vi "Request Joystick State.vi"(8 "error in (no error)":errorcluster, 9 "Caller Enqueuer":refnum<class "Message Enqueuer.lvclass">, 10 "Joystick State Msg":refnum<class "Get Joystick State Msg.lvclass">, 11 "Joystick in":refnum<class "Joystick.lvclass">) -> (0 "error out":errorcluster, 3 "Joystick out":refnum<class "Joystick.lvclass">)   [LabVIEW 2014, in "Joystick.lvlib" / "Joystick.lvclass"]
uses:
  Joystick.lvclass
  Joystick Messages/Get Joystick State Msg/Get Joystick State Msg.lvclass
  <vilib>/ActorFramework/Message Enqueuer/Message Enqueuer.lvclass
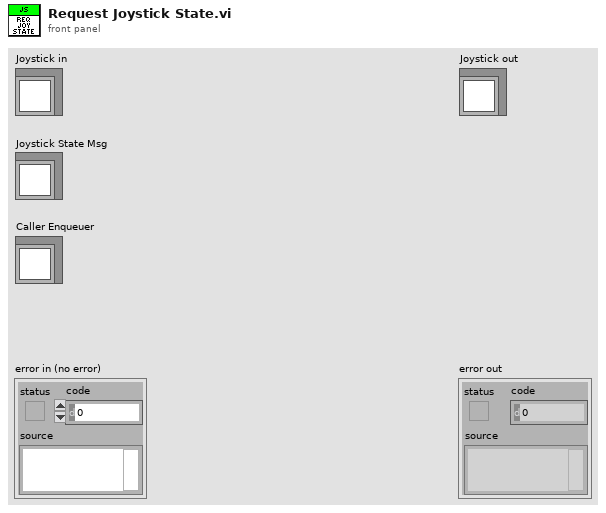
[diagram p1: front panel]
types:
  T1 = typedef "Joystick.lvlib/Joystick.lvclass/Joystick State.ctl" = cluster{"Buttons":T2[], "Axis":T3[]}
  T2 = typedef "Joystick.lvlib/Joystick.lvclass/Button State.ctl" = cluster{"Pressed":bool, "Instance Name":string, "Toggled":bool, "Just Changed":bool}
  T3 = typedef "Joystick.lvlib/Joystick.lvclass/Axis State.ctl" = cluster{"Instance Name":string, "Deadband":dbl, "Value":dbl, "At Home":bool, "Postive Axis Button State":T2, "Negative Axis Button State":T2, "Home Axis Button State":T2}
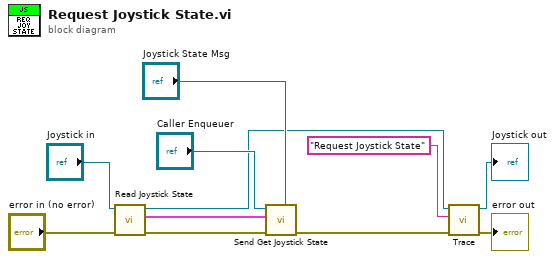
[diagram p0: block diagram]
diagram:
  n1 = call-dynamic "Read Joystick State.vi"("error in (no error)"="error in (no error)", "Joystick in"="Joystick in") -> ("error out"=w8:errorcluster, "Joystick State"=w9:T1, "Joystick out"=w3:refnum<class "Joystick.lvclass">)  [unwired: 7 in]
  n2 = call "Send Get Joystick State.vi"("Joystick.lvlib:Get Joystick State Msg.lvclass"="Joystick State Msg", "error in (no error)"=w8, "Joystick State"=w9, "Message Enqueuer"="Caller Enqueuer") -> ("error out"=w5:errorcluster)  [unwired: 6 in, 1 out]
  n3 = call-dynamic "Trace.vi"("error in (no error)"=w5, "System Action"="Request Joystick State", "System Actor in"=w3) -> ("error out"=→"error out":errorcluster, "System Actor out"=→"Joystick out":refnum<class "Joystick.lvclass">)  [unwired: 7 in]
